vi "Check Script Checks.vi"(8 "error in (no error)":errorcluster, 11 "Tamer in":refnum<class "Tamer.lvclass">) -> (0 "error out":errorcluster, 1 "Send Result?":bool, 2 "Script Checker Result":T1, 3 "Tamer out":refnum<class "Tamer.lvclass">)   [LabVIEW 2020, in "TALOS.lvlib" / "Tamer.lvlib" / "Tamer.lvclass"]
uses:
  Tamer.lvclass
  Run Utilities/TypeDefs/Script Checker Result.ctl
  Tamer.lvclass/Tamer.ctl
  Ancestor/Ancestor/Ancestor.lvclass/Ancestor.ctl
  2654d3f6-bdb2-43f8-897d-099277a7781e.vi
  cfdf3db1-198a-4806-94d0-0758e13fc1c7.vi
  FGV/Error Memory/Get Error Description.vi
  Support VIs/Get PC name.vi
  Ancestor/Ancestor/Read ID.vi
  Support VIs/Get Class Name.vi
  <vilib>/Utility/error.llb/Clear Errors.vi
  FGV/Error Memory/Error Memory Core.vi
  <vilib>/AdvancedString/Delimited String to 1D String Array.vi
  Support VIs/Circus Root Path.vi
  FGV/Error Memory/Error Crt Lvl checker.vi
  FGV/Error Memory/Error Memory Core.vi/40c8088d-b597-4017-91af-faa98e00292e.vi
  FGV/Error Memory/Error Memory Core.vi/d4a3ab98-063c-4e44-b43d-fbdcfe6c2be2.vi
  Support VIs/Global Memory.vi
  <vilib>/Utility/LVClass/Get LV Class Name.vi
  Support VIs/Is in Packed Library.vi
  Support VIs/TALOS Root path.vi
  Support VIs/Read CSV worksheet.vi
  Support VIs/Global Constants.vi
  <vilib>/Utility/error.llb/General Error Handler.vi
  <vilib>/Comparison/Less/Less Functor/Less Functor.lvclass
  Ancestor/Ancestor/Ancestor.lvclass
  <vilib>/Comparison/Equal/Equal Functor/Equal Functor.lvclass
  TALOS.lvlib
  Run Utilities/Run Utilities.lvlib
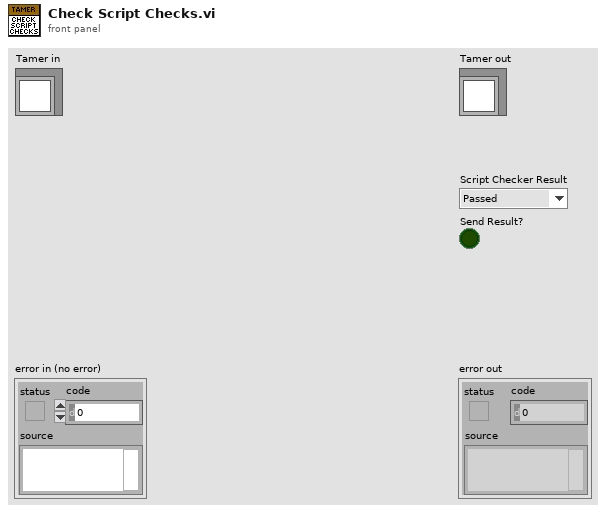
[diagram p1: front panel]
types:
  T1 = typedef "TALOS.lvlib/Run Utilities.lvlib/Script Checker Result.ctl" = enum16{"Passed", "Failed", "Empty"}
  T2 = typedef "TALOS.lvlib/Run Utilities.lvlib/Script Checker Message.ctl" = cluster{"Monkey ID":string, "Script Checker Result":T1}
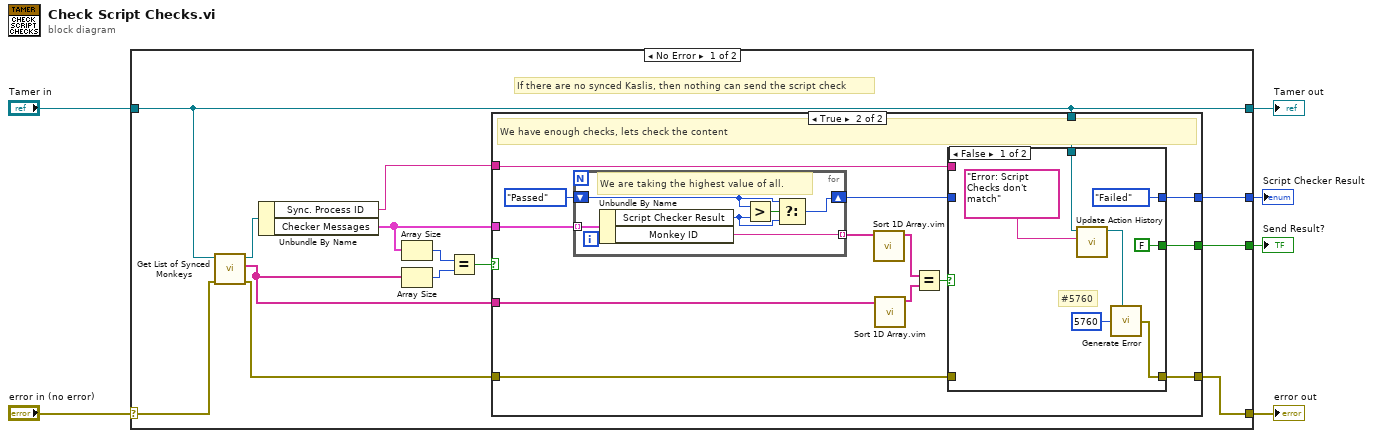
[diagram p0: block diagram]
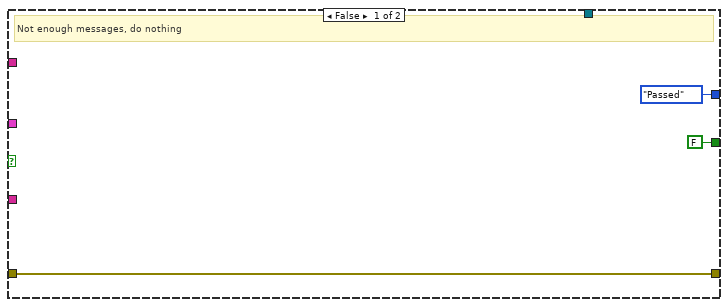
[diagram p2: hidden frame]
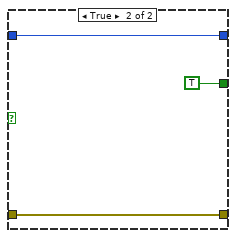
[diagram p3: hidden frame]
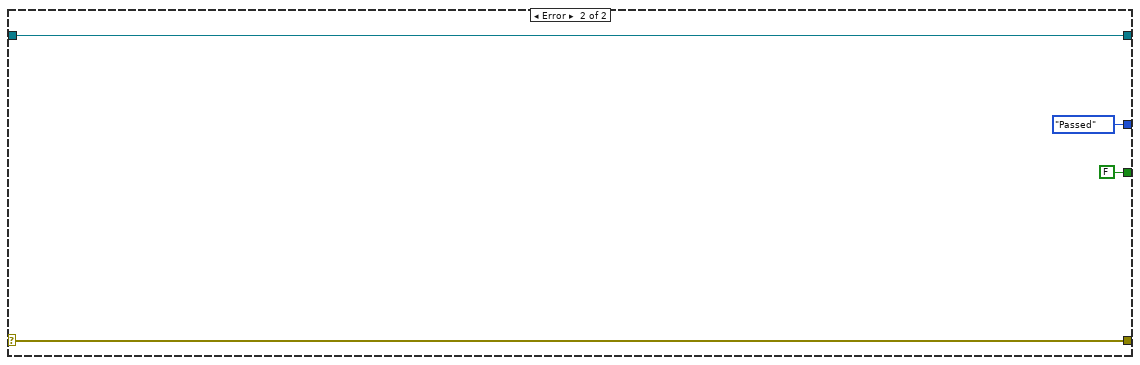
[diagram p4: hidden frame]
diagram:
  n1 = case shown="No Error" "error in (no error)" {
    selector: "error in (no error)" -> [w19 w56]
    tunnel: [w10 w56] -> w5
    tunnel: [w12 w55] -> w3
    tunnel: "Tamer in" -> [w12 w55]
    tunnel: [w8 Script_Checker_Result."Passed" ("y")] -> w2
    tunnel: [w7 FALSE] -> w1
    frame No Error {
      # "If there are no synced Kaslis, then nothing can send the script check"
      n2 = call-dynamic "Get List of Synced Monkeys.vi"("error in (no error)"=w19, "Tamer in"=w12) -> ("error out"=w11:errorcluster, "Synced Monkeys"=w13:string[], "Tamer out"=w18:refnum<class "Tamer.lvclass">)  [unwired: 7 in]
      n3 = Unbundle By Name(w18) -> ("Sync. Process ID"=w9:string, "Checker Messages"=w14:T2[])
      n4 = Array Size(array=w14) -> (size(s)=w17:i32)
      n5 = Array Size(array=w13) -> (size(s)=w16:i32)
      n6 = Equal?(x=w17, y=w16) -> (x = y?=w15:bool)
      n7 = case shown="True" w15 {
        tunnel: w14 -> [_ w36]
        tunnel: w13 -> [_ w33]
        tunnel: w12 -> [_ w28]
        tunnel: w11 -> [w22 w27]
        tunnel: [w22 w25] -> w10
        tunnel: w9 -> [_ w26]
        tunnel: [Script_Checker_Result."Passed" ("y") w24] -> w8
        tunnel: [FALSE w23] -> w7
        frame False {
          # "Not enough messages, do nothing"
        }
        frame True {
          # "We have enough checks, lets check the content"
          n8 = for {
            tunnel: w36 -> [w52] mode=indexing
            shift-right: [w50] -> w29
            shift-left: Script_Checker_Result."Passed" ("y") -> [w48]
            tunnel: [w47] -> w34 mode=indexing
            # "We are taking the highest value of all."
            n9 = Unbundle By Name(w52) -> ("Script Checker Result"=w49:T1, "Monkey ID"=w47:string)
            n10 = Greater?(x=w48, y=w49) -> (0:w51:bool)
            n11 = Select(t=w48, s=w51, f=w49) -> (s? t:f=w50:T1)
          }
          n12 = call "Sort 1D Array.vim"("unsorted array"=w34) -> ("sorted array"=w31:string[])  [unwired: 10 in]
          n13 = call "Sort 1D Array.vim"("unsorted array"=w33) -> ("sorted array"=w32:string[])  [unwired: 10 in]
          n14 = Equal?(x=w31, y=w32) -> (x = y?=w30:bool)
          n15 = case shown="False" w30 {
            tunnel: w29 -> [_ w45]
            tunnel: w28 -> [w41 _]
            tunnel: w27 -> [_ w46]
            tunnel: [w39 w46] -> w25
            tunnel: w26 -> [_ _]
            tunnel: [Script_Checker_Result."Failed" ("y") w45] -> w24
            tunnel: [FALSE TRUE] -> w23
            frame False {
              # "#5760"
              n16 = call-dynamic "Update Action History.vi"("Action"="Error: Script Checks don't match", "Tamer in"=w41) -> ("Tamer out"=w40:refnum<class "Tamer.lvclass">)  [unwired: 8 in, 1 out]
              n17 = call "Generate Error.vi"("Class"=w40, "Error Code"=5760) -> ("error out"=w39:errorcluster)  [unwired: 5 in]
            }
            frame True {
            }
          }
        }
      }
    }
    frame Error {
    }
  }
  "error out" <- w5
  "Tamer out" <- w3
  "Script Checker Result" <- w2
  "Send Result?" <- w1
